vi "ExtractDataFromXML.vi"(8 "error in (no error)":errorcluster, 11 "path to XML document":path) -> (0 "error out":errorcluster, 3 "XML Data":T1[](array[typedef]))   [LabVIEW 2020]
uses:
  <vilib>/regexp/Match Regular Expression.xnode
  <vilib>/xml/NI_XML.lvlib
  <vilib>/xml/Load XML File.vi
  <resource>/objmgr/DOMUserDefRef.rc
  <vilib>/xml/Close Reference(Node).vi
  <vilib>/xml/Close Reference(NdList).vi
  Controls/XMLDataStructureIconLibrary.ctl
panel:
  in  "XML Data":T1
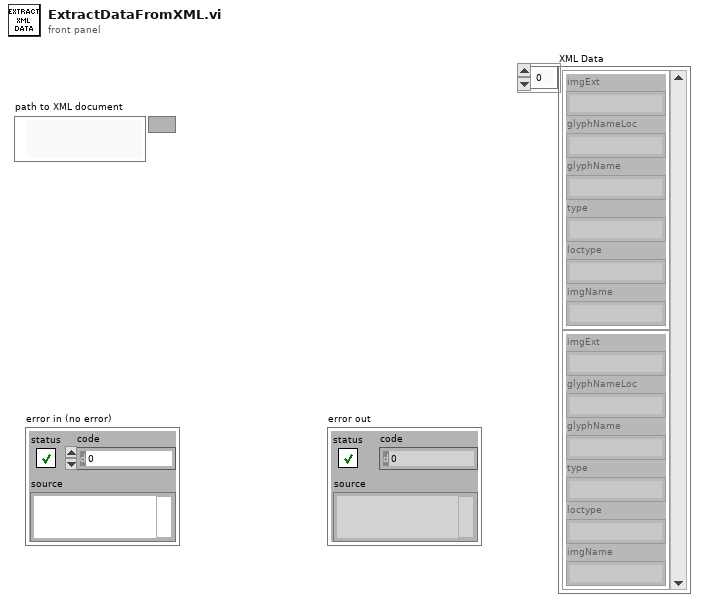
[diagram p1: front panel]
types:
  T1 = typedef "XMLDataStructureIconLibrary.ctl" = cluster{"imgExt":string, "glyphNameLoc":string, "glyphName":string, "type":string, "loctype":string, "imgName":string}
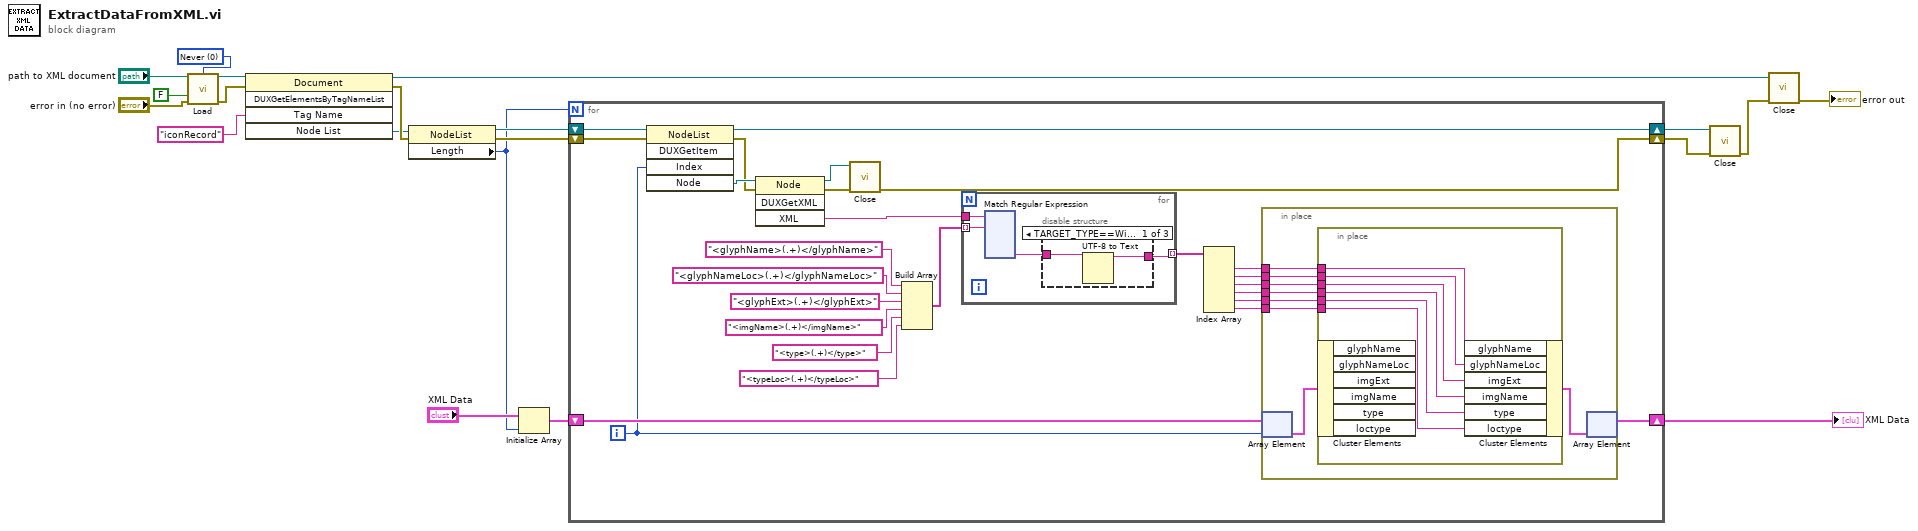
[diagram p0: block diagram]
diagram:
  w18 = 0 items=["Never", "Always", "Auto"] ("validate on load (Auto)")
  n1 = call-poly <vilib>:"Load.vi"("path to XML document"="path to XML document", "validate on load (Auto)"=w18, "load external DTD (True)"=FALSE, "error in (no error)"="error in (no error)") -> ("DOM document out"=w15:refnum<k20>, "error out"=w14:errorcluster)  [unwired: 9 in, 1 out]
  n2 = invoke class="Document" method="DUXGetElementsByTagNameList"(reference=w15, error in=w14, "Tag Name"="iconRecord") -> (reference out=w13:refnum<k20>, error out=w10:errorcluster, "Node List"=w9:refnum<k20>)  [unwired: 2 in, 2 out]
  n3 = property class="NodeList"(reference=w9, error in=w10) -> (reference out=w8:refnum<k20>, error out=w7:errorcluster, "Length"=w2:i32)
  n4 = Initialize Array("XML Data", w2) -> (w4:T1[])
  n5 = for {
    N: w2 -> [_]
    shift-right: [w30] -> w6
    shift-left: w7 -> [w44]
    shift-right: [w31] -> w5
    shift-left: w8 -> [w43]
    shift-right: [w45] -> w11
    shift-left: w4 -> [w46]
    i -> [w42]
    n6 = invoke class="NodeList" method="DUXGetItem"(reference=w43, error in=w44, "Index"=w42) -> (reference out=w31:refnum<k20>, error out=w40:errorcluster, "Node"=w41:refnum<k20>)  [unwired: 2 in, 2 out]
    n7 = invoke class="Node" method="DUXGetXML"(reference=w41, error in=w40) -> (reference out=w32:refnum<k20>, error out=w29:errorcluster, "XML"=w21:string)  [unwired: 2 in, 1 out]
    n8 = call-poly <vilib>:"Close.vi"("error in (no error)"=w29, "node"=w32) -> ("error out"=w30:errorcluster)  [unwired: 7 in]
    n9 = Build Array("<glyphName>(.+)</glyphName>" ("regular expression"), "<glyphNameLoc>(.+)</glyphNameLoc>" ("regular expression"), "<glyphExt>(.+)</glyphExt>" ("regular expression"), "<imgName>(.+)</imgName>" ("regular expression"), "<type>(.+)</type>" ("regular expression"), "<typeLoc>(.+)</typeLoc>" ("regular expression")) -> (w33:string[])
    n10 = for {
      tunnel: w33 -> [w50] mode=indexing
      tunnel: [w47] -> w28 mode=indexing
      tunnel: w21 -> [w49]
      n11 = xnode "Match Regular Expression"("input string"=w49, "regular expression"=w50) -> ("submatch 1"=w48:string)  [unwired: 4 in, 5 out]
      n12 = disable-structure shown="TARGET_TYPE==Windows, default" {
        disable-tunnel: w48 -> [w52 w53 w54]
        disable-tunnel: [w51 w53 w54] -> w47
        frame condition #0 (active) {
          n13 = UTF-8 to Text(11:w52) -> (3:w51:string)  [unwired: 2 in, 1 out]
        }
        frame condition #1 {
        }
        frame condition #2 {
        }
      }
    }
    n14 = Index Array(array=w28) -> (element #1=w27:string, element #2=w26:string, element #3=w25:string, element #4=w24:string, element #5=w23:string, element #6=w22:string)  [unwired: 6 in]
    n15 = in-place {
      in-place-border: w27 -> [w179]
      in-place-border: w26 -> [w178]
      in-place-border: w25 -> [w177]
      in-place-border: w24 -> [w176]
      in-place-border: w23 -> [w175]
      in-place-border: w22 -> [w174]
      n16 = in-place-array #1(w46, w42) -> (w181:T1)
      n17 = in-place {
        in-place-border: w179 -> [w187]
        in-place-border: w178 -> [w186]
        in-place-border: w177 -> [w185]
        in-place-border: w176 -> [w184]
        in-place-border: w175 -> [w183]
        in-place-border: w174 -> [w182]
        n18 = in-place-cluster #2(w181) -> ()  [unwired: 6 out]
        n19 = in-place-cluster #2("glyphName"=w187, "glyphNameLoc"=w186, "imgExt"=w185, "imgName"=w184, "type"=w183, "loctype"=w182) -> (w180:T1)
      }
      n20 = in-place-array #1(w180) -> (w45:T1[])  [unwired: 1 out]
    }
  }
  "XML Data" <- w11
  n21 = call-poly <vilib>:"Close.vi"("error in (no error)"=w6, "node list"=w5) -> ("error out"=w12:errorcluster)  [unwired: 7 in]
  n22 = call-poly <vilib>:"Close.vi"("error in (no error)"=w12, "node"=w13) -> ("error out"=→"error out":errorcluster)  [unwired: 7 in]
